vi "Refresh Settings.vi"(8 "error in":errorcluster, 11 "PRM in":refnum<class "PRM.lvclass">) -> (0 "error out":errorcluster, 3 "PRM out":refnum<class "PRM.lvclass">)   [LabVIEW 2019, in "PRM.lvlib" / "PRM.lvclass"]
uses:
  Library/PRM.lvclass
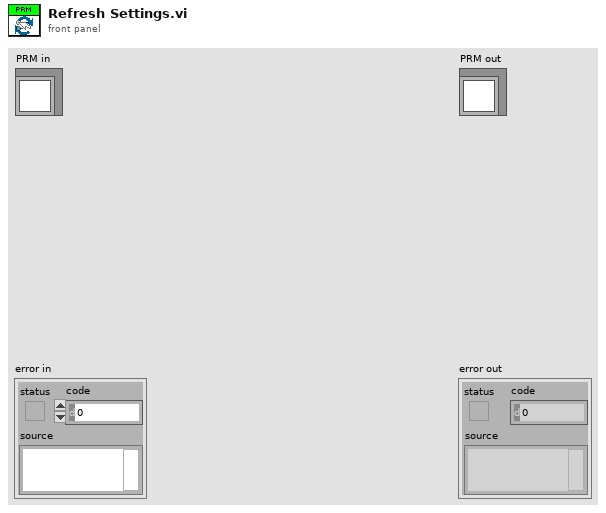
[diagram p1: front panel]
types:
  T1 = typedef "PRM.lvlib/PRM.lvclass/Operational Mode.ctl" = enum16{"RESISTANCE", "TEMPERATURE", "POTENTIOMETER"}
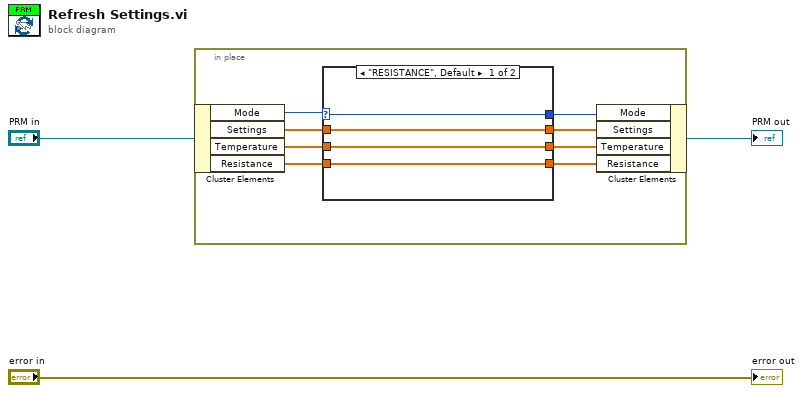
[diagram p0: block diagram]
diagram:
  n1 = in-place {
    n2 = in-place-cluster #1("PRM in") -> ("Mode"=w11:T1, "Settings"=w9:dbl[], "Temperature"=w7:dbl[], "Resistance"=w5:dbl[])
    n3 = case shown="\"RESISTANCE\", Default" w11 {
      selector: w11 -> [w15 w18]
      tunnel: [w15 w18] -> w10
      tunnel: w9 -> [w14 w17]
      tunnel: [w14 w17] -> w8
      tunnel: w7 -> [w13 _]
      tunnel: [w13 w17] -> w6
      tunnel: w5 -> [w12 w16]
      tunnel: [w12 w16] -> w4
      frame "RESISTANCE", Default {
      }
      frame "TEMPERATURE" {
      }
    }
    n4 = in-place-cluster #1("Mode"=w10, "Settings"=w8, "Temperature"=w6, "Resistance"=w4) -> (→"PRM out":refnum<class "PRM.lvclass">)
  }
  "error out" <- "error in"
